vi "center of circle.vi"(9 "point 3":dbl[](array[numeric]), 10 "point 2":dbl[](array[numeric]), 11 "point 1":dbl[](array[numeric])) -> (2 "y coord":dbl, 3 "x coord":dbl)   [LabVIEW 2011]
uses:
  <vilib>/Analysis/7linalg.llb/Solve Linear Equations (single right hand).vi
  <vilib>/Analysis/7linalg.llb/Solve Linear Eqs (General).vi
  <vilib>/Analysis/7linalg.llb/Solve Linear Eqs (Gen, single right hand).vi
  <vilib>/Analysis/NI_AALPro.lvlib
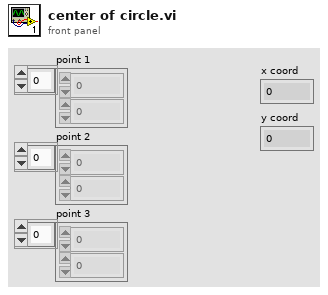
[diagram p1: front panel]
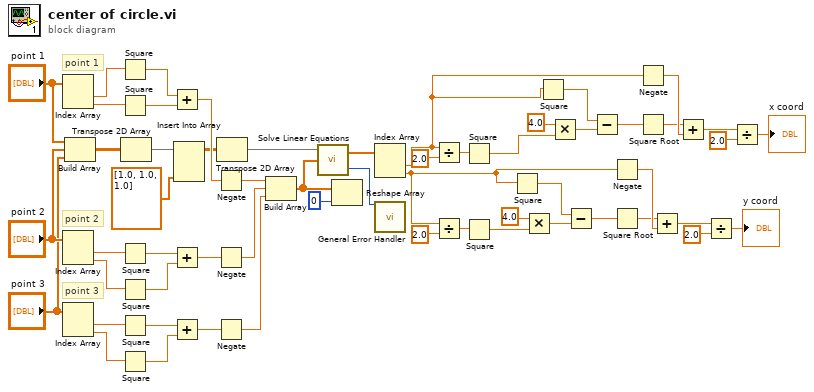
[diagram p0: block diagram]
diagram:
  # "point 3"
  # "point 2"
  # "point 1"
  n1 = Index Array(array="point 1") -> (element #1=w53:dbl, element #2=w55:dbl)  [unwired: 2 in]
  n2 = Index Array(array="point 2") -> (element #1=w48:dbl, element #2=w50:dbl)  [unwired: 2 in]
  n3 = Index Array(array="point 3") -> (element #1=w43:dbl, element #2=w45:dbl)  [unwired: 2 in]
  n4 = Build Array("point 1", "point 2", "point 3") -> (w33:dbl[][])
  n5 = Square(x=w53) -> (x^2=w52:dbl)
  n6 = Square(x=w55) -> (x^2=w54:dbl)
  n7 = Square(x=w48) -> (x^2=w47:dbl)
  n8 = Square(x=w50) -> (x^2=w49:dbl)
  n9 = Square(x=w43) -> (x^2=w42:dbl)
  n10 = Square(x=w45) -> (x^2=w44:dbl)
  n11 = Transpose 2D Array(2D array=w33) -> (transposed array=w32:dbl[][])
  n12 = Add(x=w52, y=w54) -> (x+y=w51:dbl)
  n13 = Add(x=w47, y=w49) -> (x+y=w46:dbl)
  n14 = Add(x=w42, y=w44) -> (x+y=w41:dbl)
  n15 = Insert Into Array(array=w32, new element=dbl[] [1.0, 1.0, 1.0] ("new element/subarray")) -> (w29:dbl[][])  [unwired: 2 in]
  n16 = Negate(x=w51) -> (-x=w38:dbl)
  n17 = Negate(x=w46) -> (-x=w37:dbl)
  n18 = Negate(x=w41) -> (-x=w36:dbl)
  n19 = Transpose 2D Array(2D array=w29) -> (transposed array=w28:dbl[][])
  n20 = Build Array(w38, w37, w36) -> (w31:dbl[])
  n21 = call-poly <vilib>:"Solve Linear Equations.vi"("Known Vector"=w31, "Input Matrix"=w28) -> ("error"=w35:i32, "Solution Vector"=w27:dbl[])  [unwired: 1 in]
  n22 = Reshape Array(w31, 0 ("dimension size")) -> ()  [unwired: 1 out]
  n23 = Index Array(array=w27) -> (element #1=w1:dbl, element #2=w20:dbl)  [unwired: 2 in]
  n24 = call <vilib>:"General Error Handler.vi"("[error code] (0)"=w35) -> ()  [unwired: 10 in, 5 out]
  n25 = Divide(x=w1, y=2.0) -> (x/y=w25:dbl)
  n26 = Divide(x=w20, y=2.0) -> (x/y=w23:dbl)
  n27 = Square(x=w25) -> (x^2=w2:dbl)
  n28 = Square(x=w23) -> (x^2=w17:dbl)
  n29 = Square(x=w20) -> (x^2=w19:dbl)
  n30 = Multiply(x=4.0, y=w17) -> (x*y=w16:dbl)
  n31 = Square(x=w1) -> (x^2=w9:dbl)
  n32 = Multiply(x=4.0, y=w2) -> (x*y=w7:dbl)
  n33 = Subtract(x=w19, y=w16) -> (x-y=w15:dbl)
  n34 = Subtract(x=w9, y=w7) -> (x-y=w6:dbl)
  n35 = Negate(x=w20) -> (-x=w22:dbl)
  n36 = Square Root(x=w15) -> (sqrt(x)=w21:dbl)
  n37 = Negate(x=w1) -> (-x=w11:dbl)
  n38 = Square Root(x=w6) -> (sqrt(x)=w10:dbl)
  n39 = Add(x=w21, y=w22) -> (x+y=w14:dbl)
  n40 = Add(x=w10, y=w11) -> (x+y=w5:dbl)
  n41 = Divide(x=w14, y=2.0) -> (x/y=→"y coord":dbl)
  n42 = Divide(x=w5, y=2.0) -> (x/y=→"x coord":dbl)
